vi "UI Initialize Device.vi"(8 "error in":errorcluster) -> (0 "error out":errorcluster)   [LabVIEW 2019, in "Initialize.lvlib"]
uses:
  Initialize.lvlib
  Queues/Message Cluster.ctl
  <vilib>/Utility/miscctls.llb/LVPointTypeDef.ctl
  Fluidic Process/SubVI/Fluidic Para.ctl
  LED/SubVI/Image Para.ctl
  Camera/Andor/SubVI/seletion.ctl
  <vilib>/Utility/file.llb/Read Delimited Spreadsheet (string).vi
  <vilib>/Utility/error.llb/Error Cluster From Error Code.vi
  <vilib>/ErrorRing/Error Ring.xnode
  Camera/Andor/Andor.lvlib
  IO/sbRIO9623/sbRIO9623.lvlib
  Laser/Coherent/Coherent.lvlib
  LED/LED.lvlib
  Motion/Allmotion/Allmotion.lvlib
  Selection Valve/IDEX/IDEX.lvlib
  Syringe Pump/NE-500/NE-500.lvlib
  Queues/Queues.lvlib
  Fluidic Process/Fluidic Process.lvlib
  Image/Image.lvlib
panel:
  in  "Start":bool
  in  "Operator":string
  in  "Experiment":string
  out "Homing":bool
  in  "Done":bool
  out "Syringe Pump":bool
  out "Selection Valve":bool
  out "Motion":bool
  out "LED":bool
  out "Laser":bool
  out "I/O":bool
  out "Camera":bool
  in  "Abort":bool
  in  "Next":bool
  # "Step 1. Experiment Info"
  # "Step 2. Device"
  # "Step 3. Chip"
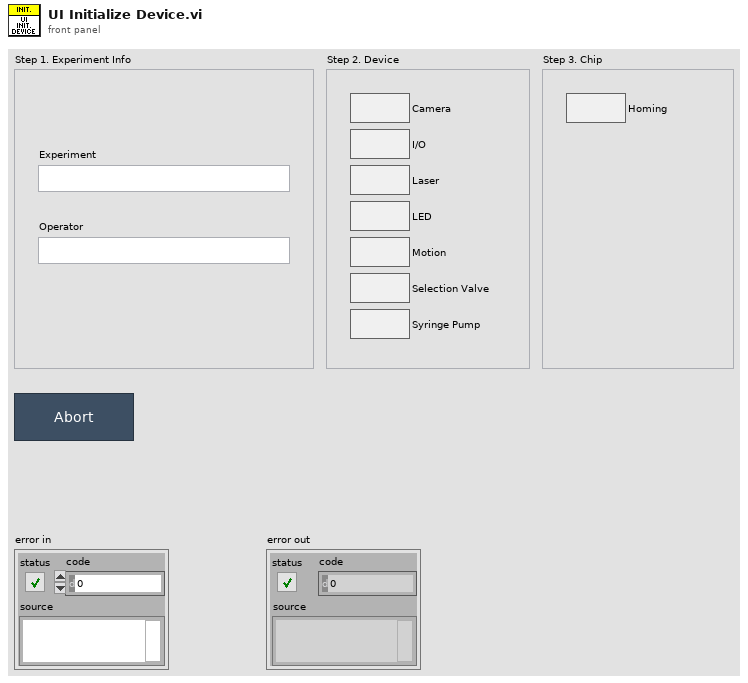
[diagram p1: front panel]
types:
  T1 = cluster{"VISA laser":refnum<visa-resource-name>, "VISA motion":refnum<visa-resource-name>, "Device Status":cluster{"Syringe Pump":bool, "Selection Valve":bool, "Motion":bool, "Camera":bool, "LED":bool, "Laser":bool, "I/O":bool}, "Tick Count":u32, "Chip Status":cluster{"Air Sealing":bool, "Homing":bool, "Locating":bool}, "Experiment":string, "Operator":string, "Folder Path":path}
  T2 = typedef "LVPointTypeDef.ctl" = cluster{"Horizontal":i16, "Vertical":i16}
  T3 = typedef "Queues.lvlib/Message Cluster.ctl" = cluster{"State":string, "Data":variant}
  T4 = typedef "Fluidic Process.lvlib/Fluidic Para.ctl" = cluster{"Read Force Sensor":i32, "Read Regulator":i32, "Read Force Sensor?":bool, "Read Regulator?":bool, "Read Syringe Pump":i32, "Read Syringe Pump?":bool}
  T5 = typedef "LED.lvlib/Image Para.ctl" = cluster{"Marker":T6, "Power(Amp)":u8, "set shutter(s)":dbl, "Cube":enum16{"1", "2", "3", "4", "5", "6", "7", "8"}}
  T6 = typedef "Andor.lvlib/seletion.ctl" = enum16{"None", "Red", "Green", "Blue", "UV", "Green Laser", "Blue-Red", "UV-Red", "BF", "UV-IR"}
  T7 = typedef "ROI Descriptor" = cluster{"Global Rectangle":i32[], "Contours":cluster{"ID":enum32{"External", "Internal"}, "Type":u32, "Coordinates":i32[]}[]}
  T8 = cluster{"Image Path":path, "Start Offset":i32, "Template Path":path, "Disable Fine Search":bool, "ROI":T7}
  T9 = typedef "Initialize.lvlib/SEQ Data.ctl" = cluster{"Folder Path":path}
  T10 = typedef "Andor.lvlib/SEQ Data.ctl" = cluster{"Initialize Sucess?":bool, "Image Ref":T11, "VI Refnum":refnum<vi>}
  T11 = typedef "IMAQ Image.ctl" = refnum<image>
  T12 = typedef "sbRIO9623.lvlib/SEQ Data.ctl" = cluster{"Lid Sensor 1":bool, "Lid Sensor 2":bool, "Laser Interlock":bool, "Buffer Tank":bool, "Wash Tank":bool, "Waste Tank":bool, "SiPM 1":fxp<+,20,5>, "SiPM 2":fxp<+,20,5>, "Initialize Success?":bool, "VI Refnum":refnum<vi>}
  T13 = typedef "Coherent.lvlib/SEQ Data.ctl" = cluster{"Initialize Success?":bool, "VI Refnum":refnum<vi>}
  T14 = typedef "LED.lvlib/SEQ Data.ctl" = cluster{"Initialize Sucess?":bool, "BL2 Regulator":dbl, "BL1 Regulator":dbl, "Blood Sensor 1":dbl, "Blood Sensor 2":dbl, "Air Pressure Sensor":dbl, "Force Snesor 1":u32, "Force Snesor 2":u32, "VI Refnum":refnum<vi>}
  T15 = typedef "Allmotion.lvlib/SEQ Data.ctl" = cluster{"Position":i32[], "Arrived?":bool, "VISA name":refnum<visa-resource-name>, "Initialize Done?":bool, "State":string, "VI Refnum":refnum<vi>, "Dichroic Position":string[]}
  T16 = typedef "IDEX.lvlib/SEQ Data.ctl" = cluster{"Position":string, "Initialize Done?":bool, "VI Refnum":refnum<vi>}
  T17 = typedef "NE-500.lvlib/SEQ Data.ctl" = cluster{"Status":string, "Initialize Done?":bool, "VI Refnum":refnum<vi>}
  T18 = typedef "Fluidic Process.lvlib/SEQ Data.ctl" = cluster{"Fluidic Process Done?":bool, "Current Process":i32, "Remaining Time":dbl, "Total Process":i32, "Air Sealing":bool, "Force Condition":bool}
  T19 = typedef "Rendezvous RefNum" = refnum<k1>
  T20 = typedef "Image.lvlib/SEQ Data.ctl" = cluster{"Acquire Done?":bool, "Focus Done?":bool, "Align Done?":bool, "No Position Match?":bool, "Best Wheel Position":string, "Match Done?":bool, "Match Score":dbl, "Focus Score":dbl, "Match Position":cluster{"x":sgl, "y":sgl}, "Flower Position":i32[]}
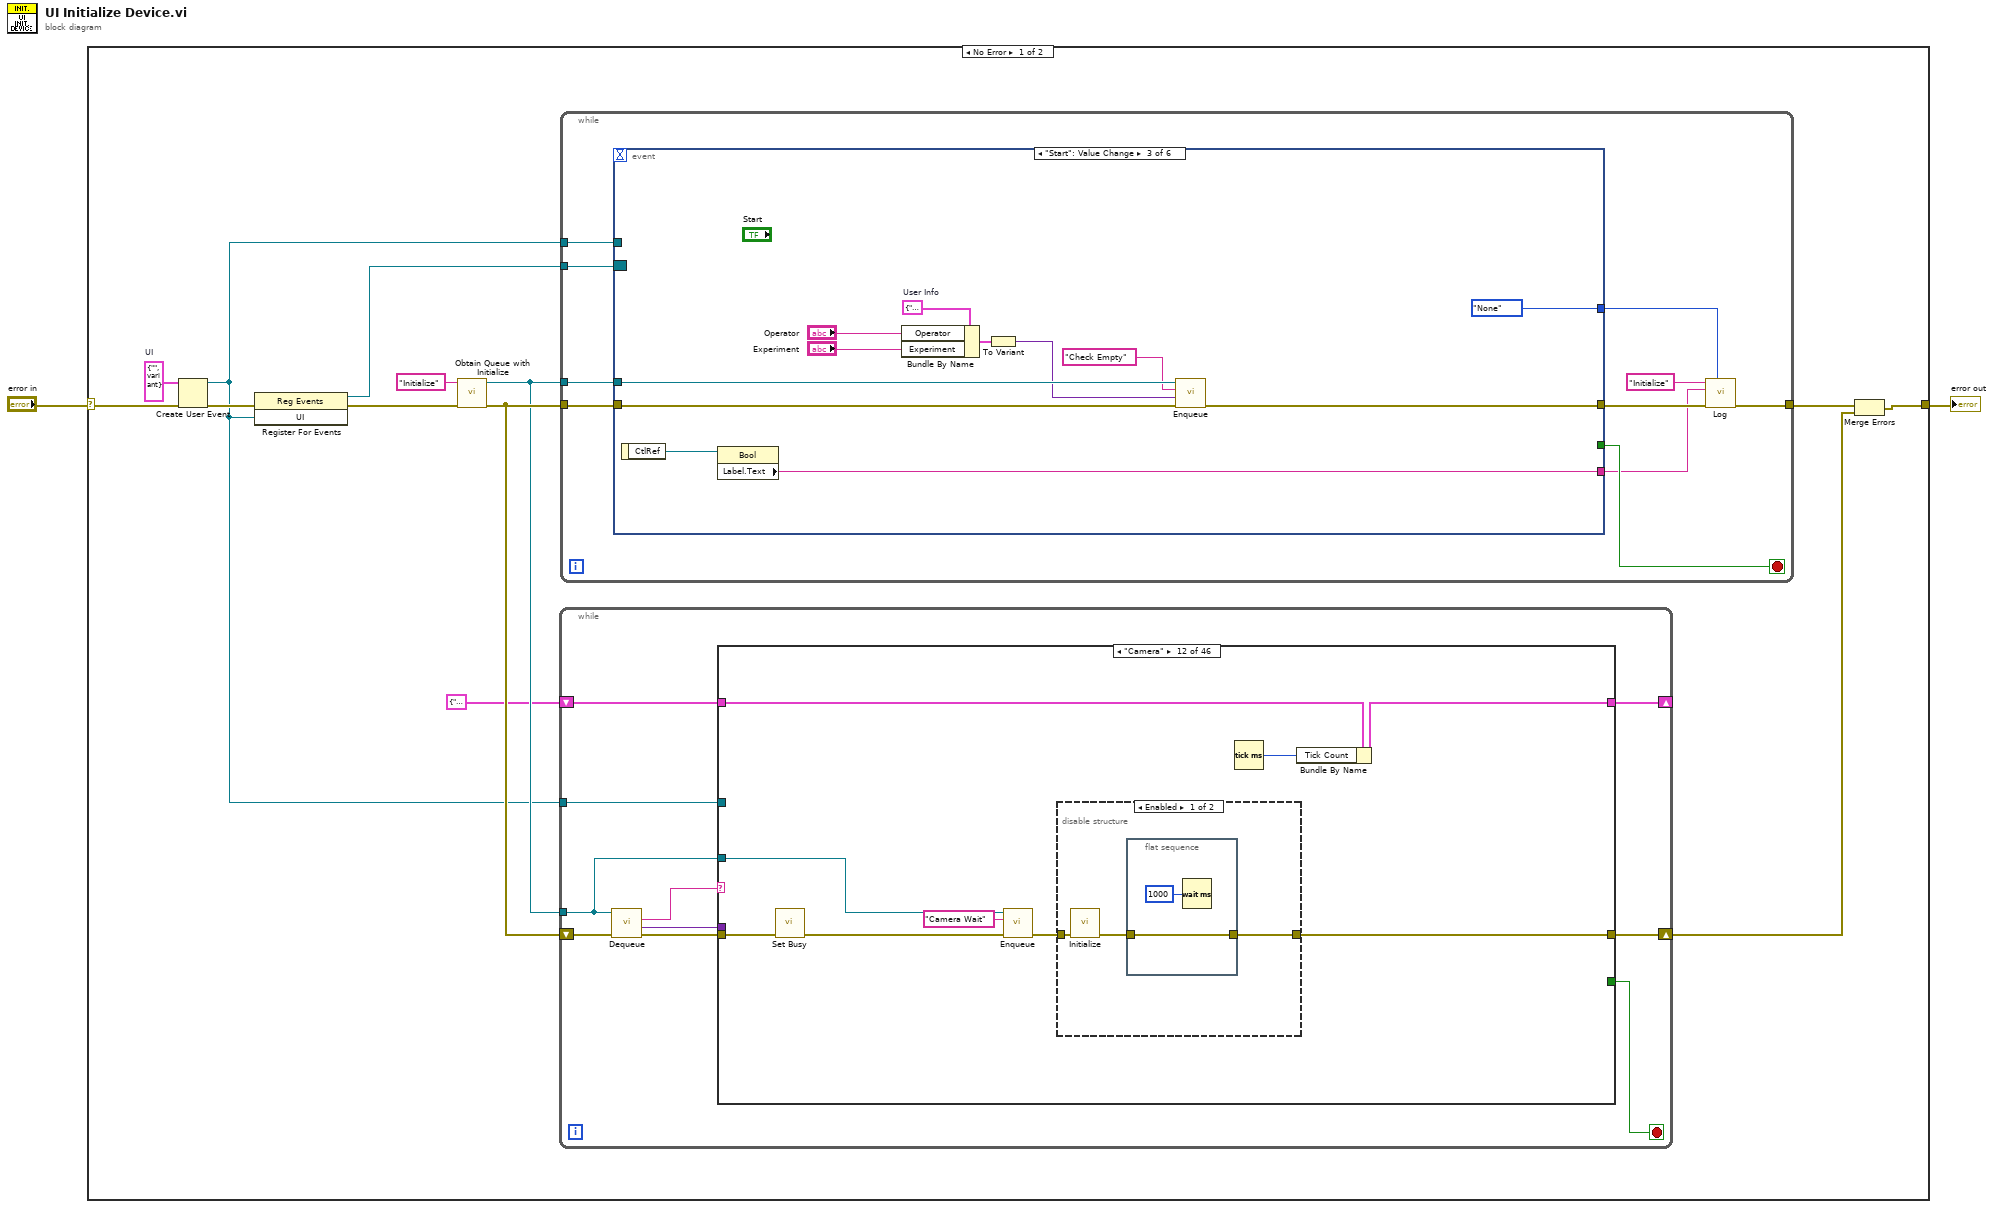
[diagram p0: block diagram]
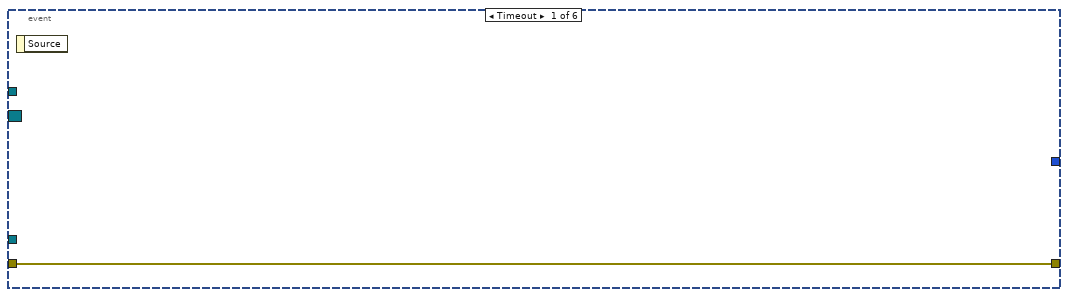
[diagram p2: hidden frame]
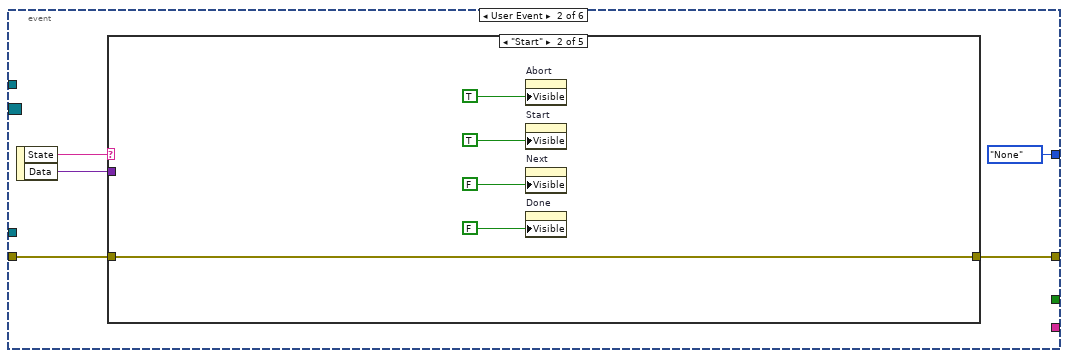
[diagram p3: hidden frame]
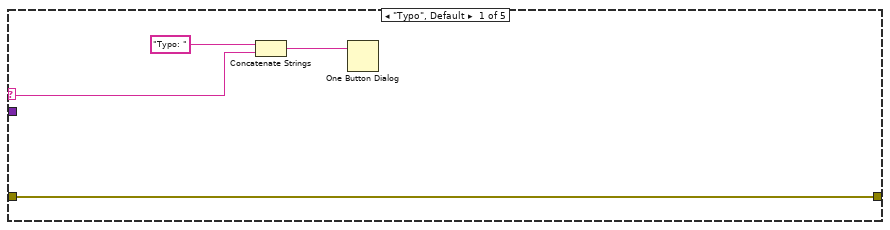
[diagram p4: hidden frame]
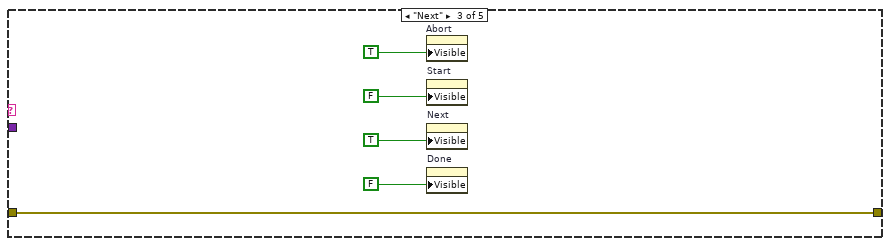
[diagram p5: hidden frame]
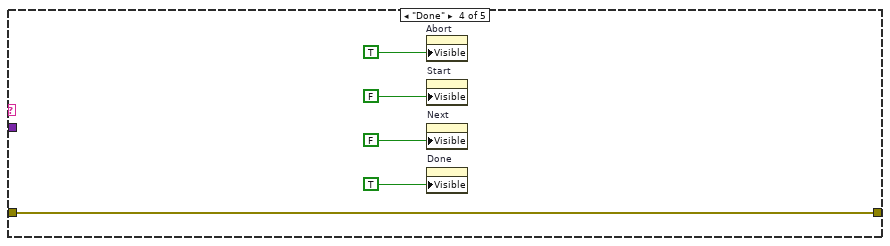
[diagram p6: hidden frame]
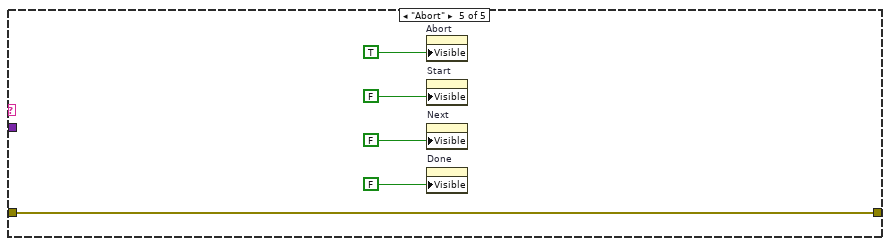
[diagram p7: hidden frame]
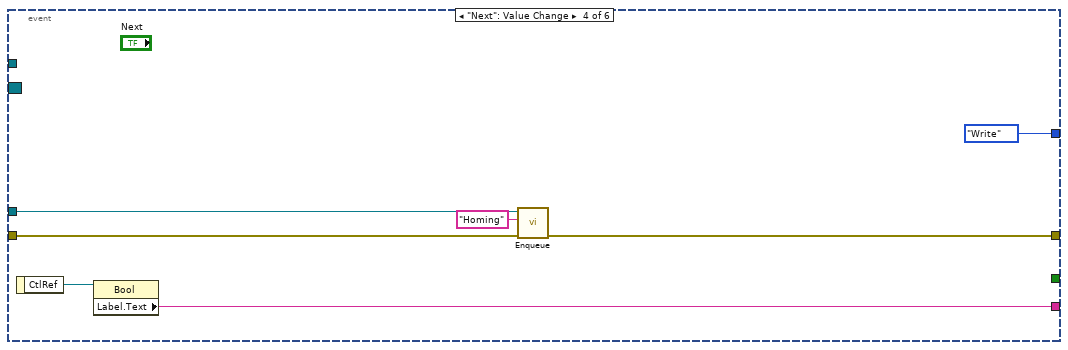
[diagram p8: hidden frame]
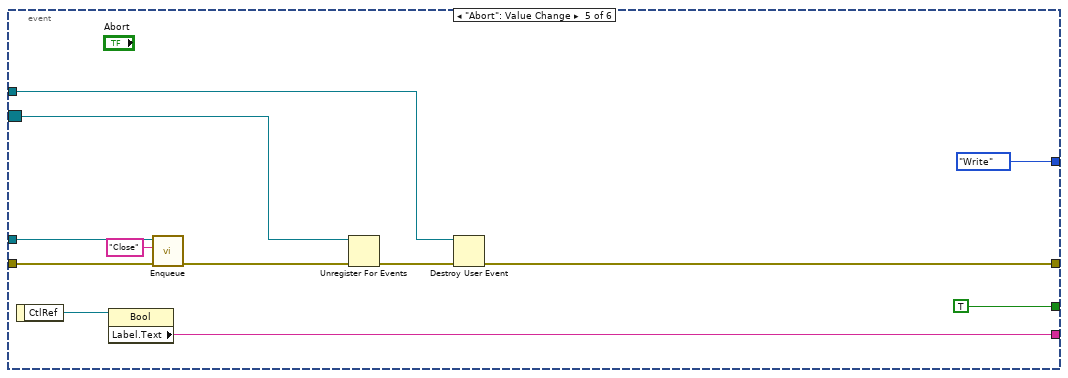
[diagram p9: hidden frame]
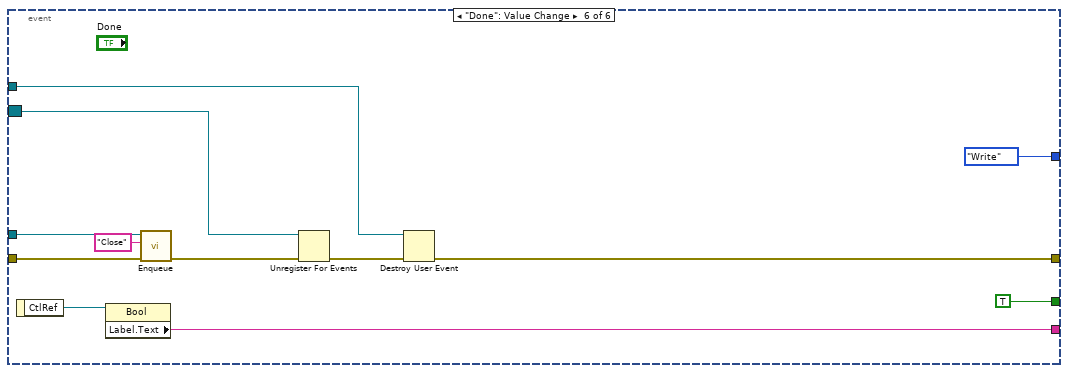
[diagram p10: hidden frame]
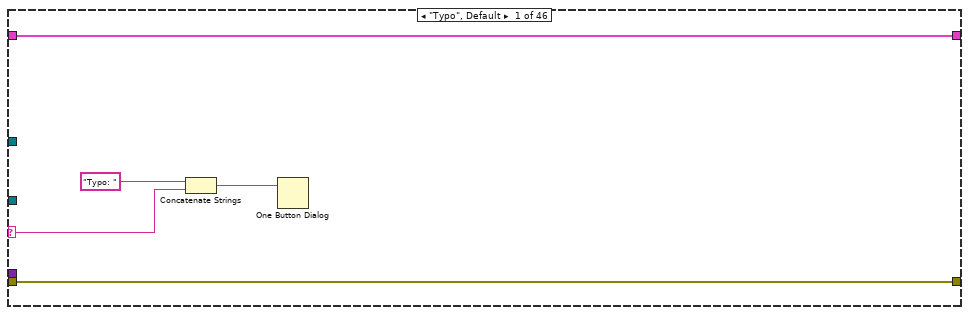
[diagram p11: hidden frame]
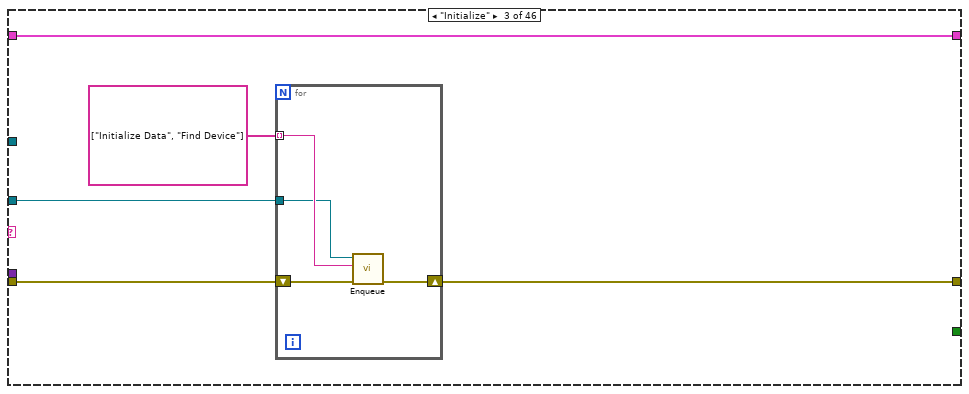
[diagram p13: hidden frame]
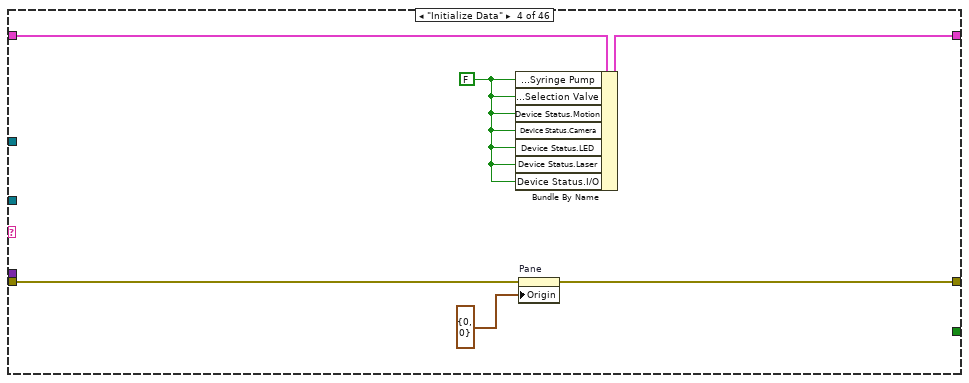
[diagram p14: hidden frame]
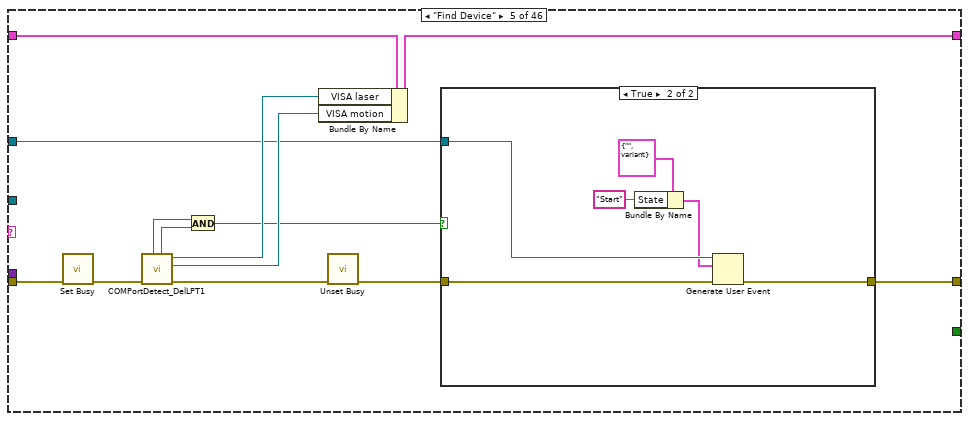
[diagram p15: hidden frame]
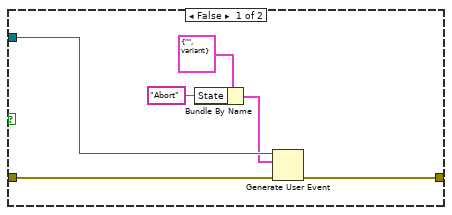
[diagram p16: hidden frame]
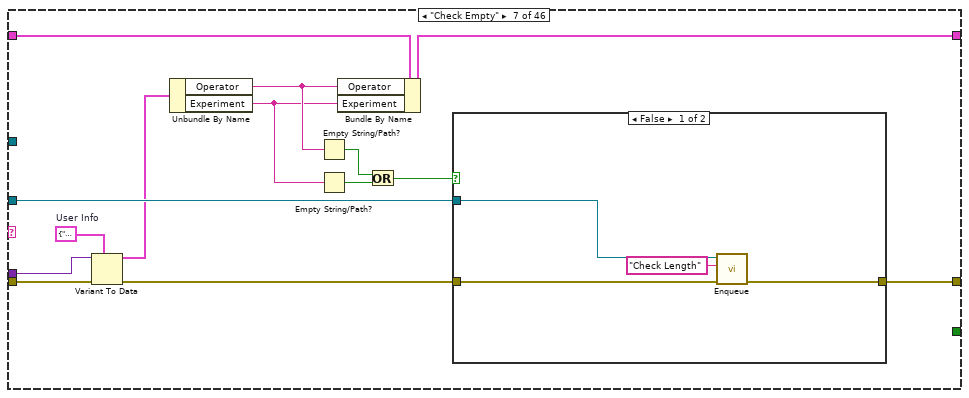
[diagram p18: hidden frame]
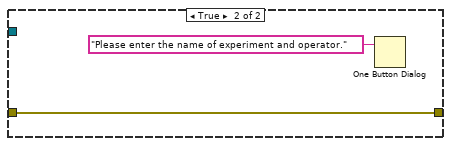
[diagram p19: hidden frame]
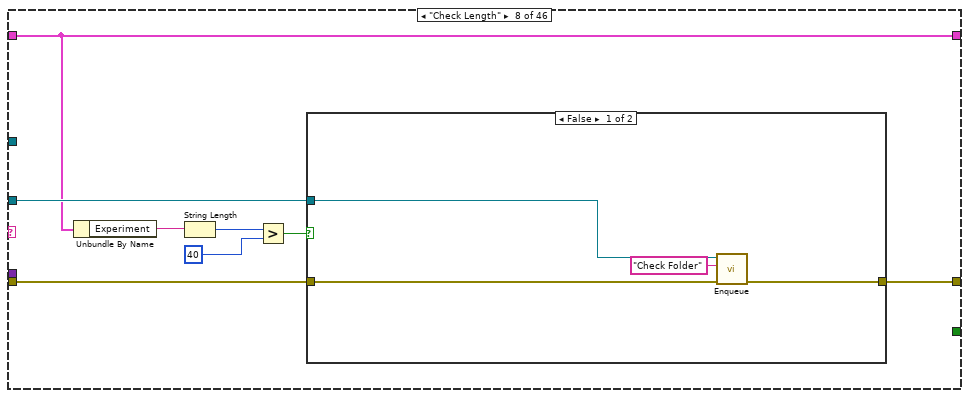
[diagram p20: hidden frame]
diagram:
  n1 = case shown="No Error" "error in" {
    selector: "error in" -> [w15 w771]
    tunnel: [w6 w771] -> w1
    frame No Error {
      w13 = T3 {"State"="", "Data"=variant}  # UI
      n2 = Create User Event(user event datatype=w13, error in=w15) -> (user event=w3:refnum<user-event>, error out=w14:errorcluster)
      n3 = register-events(error in=w14, w3) -> (reference out=w4:refnum<event-registration>, error out=w10:errorcluster)  [unwired: 1 in]
      n4 = call "Obtain Queue with Initialize.vi"("Error In"=w10, "Queue Name"="Initialize") -> ("Error Out"=w9:errorcluster, "Queue out"=w7:refnum<queue>)  [unwired: 8 in]
      n5 = while {
        tunnel: w7 -> [w104]
        shift-right: [w103] -> w11
        shift-left: w9 -> [w108]
        shift-right: [w100] -> _
        shift-left: T1 {"VISA laser"="", "VISA motion"="", "Device Status"={"Syringe Pump"=FALSE, "Selection Valve"=FALSE, "Motion"=FALSE, "Camera"=FALSE, "LED"=FALSE, "Laser"=FALSE, "I/O"=FALSE}, "Tick Count"=0, "Chip Status"={"Air Sealing"=FALSE, "Homing"=FALSE, "Locating"=FALSE}, "Experiment"="", "Operator"="", "Folder Path"=path ""} -> [w101]
        tunnel: w3 -> [w99]
        stop <- w102 stop-if-true
        n6 = call "Dequeue.vi"("Error In"=w108, "Queue in"=w104) -> ("Error Out"=w105:errorcluster, "Data"=w106:variant, "State"=w107:string)  [unwired: 6 in, 1 out]
        n7 = case shown="\"Camera\"" w107 {
          selector: w107 -> [w110 _ _ _ _ _ _ _ _ _ _ _ _ _ _ _ _ _ _ _ _ _ _ _ _ _ _ _ _ _ _ _ _ _ _ _ _ _ _ _ _ _ _ _ _ _]
          tunnel: w106 -> [_ _ _ _ _ _ w162 _ _ _ _ _ _ _ _ _ _ _ _ _ _ _ _ _ _ _ _ _ _ _ _ _ _ _ _ _ _ _ _ _ _ _ _ _ _ _]
          tunnel: w105 -> [w113 w114 w120 w127 w140 w156 w164 w183 w201 w232 w233 w236 w263 w283 w290 w317 w323 w349 w355 w382 w388 w415 w421 w448 w453 w470 w494 w503 w538 w543 w556 w578 w586 w594 w598 w629 w636 w664 w675 w704 w715 w737 w743 w747 w764 w770]
          tunnel: w104 -> [_ _ w117 _ _ _ w170 w181 w198 w231 _ w240 w254 w282 w294 w313 w327 w348 w359 w381 w392 w414 w425 w447 w457 w471 _ w501 w536 w551 w567 w577 w585 w593 w596 w628 w645 w663 w684 w703 w724 w736 w742 _ _ w769]
          tunnel: [w113 w114 w119 w126 w132 w156 w171 w182 w194 w228 w233 w242 w255 w278 w295 w314 w328 w344 w360 w375 w393 w406 w426 w439 w458 w473 w494 w498 w537 w546 w568 w572 w580 w588 w597 w624 w646 w665 w685 w705 w711 w730 w739 w750 w764 w768] -> w103
          tunnel: [_ _ _ _ _ _ _ _ _ _ _ _ _ _ _ _ _ _ _ _ _ _ _ _ _ _ _ _ _ _ _ _ _ _ _ _ _ _ _ _ _ _ _ _ _ TRUE] -> w102
          tunnel: w101 -> [w109 w115 w116 w130 w143 w157 w169 w179 w200 w224 w234 w243 w262 w280 w301 w309 w334 w341 w366 w374 w399 w410 w432 w443 w465 w481 w495 w506 w535 w549 w566 w579 w587 w595 w608 w630 w633 w659 w672 w698 w712 w738 w744 w748 w765 w766]
          tunnel: [w109 w115 w116 w129 w137 w157 w168 w179 w193 w224 w234 w238 w253 w277 w293 w311 w326 w343 w358 w379 w391 w412 w424 w445 w456 w481 w495 w497 w528 w545 w560 w579 w587 w595 w608 w623 w633 w661 w672 w701 w712 w729 w744 w748 w765 w766] -> w100
          tunnel: w99 -> [_ _ _ _ w131 _ _ _ _ _ _ _ _ _ _ _ _ _ _ _ _ _ _ _ _ w469 _ _ _ _ _ _ _ _ _ _ _ _ _ _ _ _ _ w749 _ _]
          frame "Typo", Default {
            n8 = Concatenate Strings("Typo: " ("string"), w110) -> (w112:string)
            n9 = One Button Dialog(message=w112) -> ()  [unwired: 1 in, 1 out]
          }
          frame "------Initialize------" {
          }
          frame "Initialize" {
            n10 = for {
              shift-right: [w123] -> w119
              shift-left: w120 -> [w124]
              tunnel: string[] ["Initialize Data", "Find Device"] -> [w122] mode=indexing
              tunnel: w117 -> [w121]
              n11 = call "Enqueue.vi"("Error In"=w124, "State"=w122, "Queue in"=w121) -> ("Error Out"=w123:errorcluster)  [unwired: 7 in, 1 out]
            }
          }
          frame "Initialize Data" {
            w128 = FALSE ("Initial Status.Syringe Pump")
            n12 = Bundle By Name(cluster=w130, "Device Status.Syringe Pump"=w128, "Device Status.Selection Valve"=w128, "Device Status.Motion"=w128, "Device Status.Camera"=w128, "Device Status.LED"=w128, "Device Status.Laser"=w128, "Device Status.I/O"=w128) -> (w129:T1)
            n13 = property on="Pane" class="Pane"(error in=w127, "Origin"=T2 {"Horizontal"=0, "Vertical"=0}) -> (error out=w126:errorcluster)  [unwired: 1 in, 1 out]
          }
          frame "Find Device" {
            n14 = call <vilib>:"Set Busy.vi"("error in (no error)"=w140) -> ("error out"=w139:errorcluster)  [unwired: 9 in, 1 out]
            n15 = call "COMPortDetect_DelLPT1.vi"("error in"=w139) -> ("error out"=w138:errorcluster, "VISA motion"=w135:refnum<visa-resource-name>, "VISA laser"=w136:refnum<visa-resource-name>, "Motion Find?"=w142:bool, "Laser Find?"=w141:bool)  [unwired: 6 in]
            n16 = And(x=w141, y=w142) -> (x .and. y?=w134:bool)
            n17 = Bundle By Name(cluster=w143, "VISA laser"=w136, "VISA motion"=w135) -> (w137:T1)
            n18 = call <vilib>:"Unset Busy.vi"("error in (no error)"=w138) -> ("error out"=w133:errorcluster)  [unwired: 10 in]
            n19 = case shown="True" w134 {
              tunnel: w133 -> [w149 w155]
              tunnel: [w148 w151] -> w132
              tunnel: w131 -> [w147 w154]
              frame False {
                n20 = Bundle By Name(cluster=T3 {"State"="", "Data"=variant} ("event data"), "State"="Abort") -> (w145:T3)
                n21 = Generate User Event(user event=w147, event data cluster=w145, error in=w149) -> (error out=w148:errorcluster)  [unwired: 1 in, 1 out]
              }
              frame True {
                n22 = Bundle By Name(cluster=T3 {"State"="", "Data"=variant} ("event data"), "State"="Start") -> (w152:T3)
                n23 = Generate User Event(user event=w154, event data cluster=w152, error in=w155) -> (error out=w151:errorcluster)  [unwired: 1 in, 1 out]
              }
            }
          }
          frame "------Create Folder------" {
          }
          frame "Check Empty" {
            w161 = cluster{"Operator":string, "Experiment":string} {"Operator"="", "Experiment"=""}  # User Info
            n24 = Variant To Data(error in=w164, type=w161, Variant=w162) -> (data=w160:cluster{"Operator":string, "Experiment":string}, error out=w163:errorcluster)
            n25 = Unbundle By Name(w160) -> ("Operator"=w159:string, "Experiment"=w158:string)
            n26 = Empty String/Path?(string/path=w159) -> (empty?=w167:bool)
            n27 = Empty String/Path?(string/path=w158) -> (empty?=w166:bool)
            n28 = Bundle By Name(cluster=w169, "Operator"=w159, "Experiment"=w158) -> (w168:T1)
            n29 = Or(x=w167, y=w166) -> (x .or. y?=w165:bool)
            n30 = case shown="False" w165 {
              tunnel: w163 -> [w175 w177]
              tunnel: [w174 w177] -> w171
              tunnel: w170 -> [w173 _]
              frame False {
                n31 = call "Enqueue.vi"("Error In"=w175, "State"="Check Length", "Queue in"=w173) -> ("Error Out"=w174:errorcluster)  [unwired: 7 in, 1 out]
              }
              frame True {
                n32 = One Button Dialog(message="Please enter the name of experiment and operator.") -> ()  [unwired: 1 in, 1 out]
              }
            }
          }
          frame "Check Length" {
            n33 = Unbundle By Name(w179) -> ("Experiment"=w178:string)
            n34 = String Length(string=w178) -> (length=w185:i32)
            n35 = Greater?(x=w185, y=40) -> (0:w180:bool)
            n36 = case shown="False" w180 {
              tunnel: w183 -> [w189 w191]
              tunnel: [w188 w191] -> w182
              tunnel: w181 -> [w187 _]
              frame False {
                n37 = call "Enqueue.vi"("Error In"=w189, "State"="Check Folder", "Queue in"=w187) -> ("Error Out"=w188:errorcluster)  [unwired: 7 in, 1 out]
              }
              frame True {
                n38 = One Button Dialog(message="Please limit the Sample ID to less than 40 characters and do not use spaces and symbols.") -> ()  [unwired: 1 in, 1 out]
              }
            }
          }
          frame "Check Folder" {
            n39 = Unbundle By Name(w200) -> ("Experiment"=w199:string)
            n40 = Format Date/Time String(time format string (%c)="%Y%m%d") -> (date/time string=w205:string)  [unwired: 2 in]
            n41 = Concatenate Strings(w205, "\\", w199) -> (w206:string)
            n42 = Build Path(base path=path "C:/MiCareo/MiSelect2015QQ01/DATA", name or relative path=w206) -> (appended path=w207:path)
            n43 = call <vilib>:"Check if File or Folder Exists.vi"("error in (no error)"=w201, "path"=w207) -> ("error out"=w195:errorcluster, "file or folder exists?"=w197:bool, "dup path"=w196:path)  [unwired: 7 in]
            n44 = case shown="False" w197 {
              tunnel: w198 -> [w215 _]
              tunnel: w196 -> [w208 _]
              tunnel: w195 -> [w217 w219]
              tunnel: [w216 w219] -> w194
              tunnel: [w208 _] -> w192
              frame False {
                n45 = Create Folder(path (use dialog)=w208, error in=w217) -> (error out=w213:errorcluster)  [unwired: 1 in, 2 out]
                n46 = call "SEQ Preview Queue.vi"("error in"=w213) -> ("error out"=w212:errorcluster, "SEQ Data"=w210:T9)  [unwired: 9 in]
                n47 = Bundle By Name(cluster=w210, "Folder Path"=w208) -> (w209:T9)
                n48 = call "SEQ Lossy Queue.vi"("error in"=w212, "SEQ Data"=w209) -> ("error out"=w211:errorcluster)  [unwired: 9 in]
                n49 = call "Enqueue.vi"("Error In"=w211, "State"="Write User Info", "Queue in"=w215) -> ("Error Out"=w216:errorcluster)  [unwired: 7 in, 1 out]
              }
              frame True {
                n50 = One Button Dialog(message="This name of the experiment has already been used") -> ()  [unwired: 1 in, 1 out]
              }
            }
            n51 = Bundle By Name(cluster=w200, "Folder Path"=w192) -> (w193:T1)
          }
          frame "Write User Info" {
            n52 = Unbundle By Name(w224) -> ("Operator"=w222:string, "Experiment"=w221:string)
            n53 = call "Enqueue.vi"("Error In"=w232, "State"="Camera", "Queue in"=w231) -> ("Error Out"=w229:errorcluster)  [unwired: 7 in, 1 out]
            n54 = Format Into String(format string="Operator: %s, Experiment: %s", w222, w221) -> (resulting string=w220:string)  [unwired: 2 in, 1 out]
            n55 = call "Log.vi"("Action"=enum16{"None", "Write"}."Write", "error in"=w229, "Description"=w220, "State"="User Info", "Page Name"="Initialize") -> ("error out"=w228:errorcluster)  [unwired: 6 in]
          }
          frame "------Device------" {
          }
          frame "Camera" {
            n56 = call <vilib>:"Set Busy.vi"("error in (no error)"=w236) -> ("error out"=w235:errorcluster)  [unwired: 9 in, 1 out]
            n57 = call "Enqueue.vi"("Error In"=w235, "State"="Camera Wait", "Queue in"=w240) -> ("Error Out"=w241:errorcluster)  [unwired: 7 in, 1 out]
            n58 = disable-structure shown="Enabled" {
              disable-tunnel: [w245 w249] -> w242
              disable-tunnel: w241 -> [w244 w249]
              frame Enabled {
                n59 = call "Initialize.vi"("Error In"=w244) -> ("Error Out"=w246:errorcluster)  [unwired: 10 in]
                n60 = flat-sequence {
                  tunnel: w246 -> [w247]
                  tunnel: [w247] -> w245
                  frame #0 {
                    n61 = Wait (ms)(milliseconds to wait=u32 1000) -> ()  [unwired: 1 out]
                  }
                }
              }
              frame Disabled {
              }
            }
            n62 = Tick Count (ms)() -> (millisecond timer value=w237:u32)
            n63 = Bundle By Name(cluster=w243, "Tick Count"=w237) -> (w238:T1)
          }
          frame "Camera Wait" {
            n64 = disable-structure shown="Enabled" {
              disable-tunnel: w263 -> [w267 w270]
              disable-tunnel: [w266 w270] -> w256
              disable-tunnel: [w265 TRUE ("Camera")] -> w252
              frame Enabled {
                n65 = call "SEQ Preview Queue.vi"("error in"=w267) -> ("error out"=w266:errorcluster, "SEQ Data"=w268:T10)  [unwired: 9 in]
                n66 = Unbundle By Name(w268) -> ("Initialize Sucess?"=w265:bool)
              }
              frame Disabled {
              }
            }
            "Camera" <- w252
            n67 = Unbundle By Name(w262) -> ("Tick Count"=w260:u32)
            n68 = Tick Count (ms)() -> (millisecond timer value=w261:u32)
            n69 = Subtract(x=w261, y=w260) -> (x-y=w259:u32)
            n70 = Greater Or Equal?(x=w259, y=u32 15000) -> (x >= y?=w250:bool)
            n71 = Or(x=w250, y=w252) -> (x .or. y?=w257:bool)
            n72 = Wait (ms)(milliseconds to wait=u32 100) -> ()  [unwired: 1 out]
            n73 = Bundle By Name(cluster=w262, "Device Status.Camera"=w252) -> (w253:T1)
            n74 = case shown="True" w257 {
              tunnel: ["Camera Wait" w273] -> w251
              tunnel: w250 -> [_ w272]
              frame False {
              }
              frame True {
                n75 = case shown="True" w272 {
                  tunnel: ["I/O" "Device End"] -> w273
                  frame False {
                  }
                  frame True {
                  }
                }
              }
            }
            n76 = call "Enqueue.vi"("Error In"=w256, "State"=w251, "Queue in"=w254) -> ("Error Out"=w255:errorcluster)  [unwired: 7 in, 1 out]
          }
          frame "I/O" {
            n77 = call "Enqueue.vi"("Error In"=w283, "State"="I/O Wait", "Queue in"=w282) -> ("Error Out"=w279:errorcluster)  [unwired: 7 in, 1 out]
            n78 = call "Initialize.vi"("Error In"=w279) -> ("Error Out"=w284:errorcluster)  [unwired: 10 in]
            n79 = flat-sequence {
              tunnel: w284 -> [w285]
              tunnel: [w285] -> w278
              frame #0 {
                n80 = Wait (ms)(milliseconds to wait=u32 1000) -> ()  [unwired: 1 out]
              }
            }
            n81 = Tick Count (ms)() -> (millisecond timer value=w276:u32)
            n82 = Bundle By Name(cluster=w280, "Tick Count"=w276) -> (w277:T1)
          }
          frame "I/O Wait" {
            n83 = call "SEQ Preview Queue.vi"("error in"=w290) -> ("error out"=w289:errorcluster, "SEQ Data"=w291:T12)  [unwired: 9 in]
            n84 = Unbundle By Name(w301) -> ("Tick Count"=w299:u32)
            n85 = Unbundle By Name(w291) -> ("Initialize Success?"=w288:bool)
            "I/O" <- w288
            n86 = Tick Count (ms)() -> (millisecond timer value=w300:u32)
            n87 = Subtract(x=w300, y=w299) -> (x-y=w298:u32)
            n88 = Greater Or Equal?(x=w298, y=u32 15000) -> (x >= y?=w287:bool)
            n89 = Or(x=w287, y=w288) -> (x .or. y?=w296:bool)
            n90 = Wait (ms)(milliseconds to wait=u32 100) -> ()  [unwired: 1 out]
            n91 = Bundle By Name(cluster=w301, "Device Status.I/O"=w288) -> (w293:T1)
            n92 = case shown="True" w296 {
              tunnel: ["I/O Wait" w305] -> w292
              tunnel: w287 -> [_ w304]
              frame False {
              }
              frame True {
                n93 = case shown="True" w304 {
                  tunnel: ["Laser" "Device End"] -> w305
                  frame False {
                  }
                  frame True {
                  }
                }
              }
            }
            n94 = call "Enqueue.vi"("Error In"=w289, "State"=w292, "Queue in"=w294) -> ("Error Out"=w295:errorcluster)  [unwired: 7 in, 1 out]
          }
          frame "Laser" {
            n95 = Unbundle By Name(w309) -> ("VISA laser"=w308:refnum<visa-resource-name>)
            n96 = call "Enqueue.vi"("Error In"=w317, "State"="Laser Wait", "Queue in"=w313) -> ("Error Out"=w315:errorcluster)  [unwired: 7 in, 1 out]
            n97 = call "Initialize.vi"("Error In"=w315, "VISA in"=w308) -> ("Error Out"=w316:errorcluster)  [unwired: 9 in]
            n98 = flat-sequence {
              tunnel: w316 -> [w318]
              tunnel: [w318] -> w314
              frame #0 {
                n99 = Wait (ms)(milliseconds to wait=u32 1000) -> ()  [unwired: 1 out]
              }
            }
            n100 = Tick Count (ms)() -> (millisecond timer value=w310:u32)
            n101 = Bundle By Name(cluster=w309, "Tick Count"=w310) -> (w311:T1)
          }
          frame "Laser Wait" {
            n102 = call "SEQ Preview Queue.vi"("error in"=w323) -> ("error out"=w322:errorcluster, "SEQ Data"=w324:T13)  [unwired: 9 in]
            n103 = Unbundle By Name(w334) -> ("Tick Count"=w332:u32)
            n104 = Unbundle By Name(w324) -> ("Initialize Success?"=w321:bool)
            "Laser" <- w321
            n105 = Tick Count (ms)() -> (millisecond timer value=w333:u32)
            n106 = Subtract(x=w333, y=w332) -> (x-y=w331:u32)
            n107 = Greater Or Equal?(x=w331, y=u32 15000) -> (x >= y?=w320:bool)
            n108 = Or(x=w320, y=w321) -> (x .or. y?=w329:bool)
            n109 = Wait (ms)(milliseconds to wait=u32 100) -> ()  [unwired: 1 out]
            n110 = Bundle By Name(cluster=w334, "Device Status.Laser"=w321) -> (w326:T1)
            n111 = case shown="True" w329 {
              tunnel: ["Laser Wait" w338] -> w325
              tunnel: w320 -> [_ w337]
              frame False {
              }
              frame True {
                n112 = case shown="True" w337 {
                  tunnel: ["LED" "Device End"] -> w338
                  frame False {
                  }
                  frame True {
                  }
                }
              }
            }
            n113 = call "Enqueue.vi"("Error In"=w322, "State"=w325, "Queue in"=w327) -> ("Error Out"=w328:errorcluster)  [unwired: 7 in, 1 out]
          }
          frame "LED" {
            n114 = call "Enqueue.vi"("Error In"=w349, "State"="LED Wait", "Queue in"=w348) -> ("Error Out"=w345:errorcluster)  [unwired: 7 in, 1 out]
            n115 = call "Initialize.vi"("Error In"=w345) -> ("Error Out"=w346:errorcluster)  [unwired: 10 in]
            n116 = flat-sequence {
              tunnel: w346 -> [w350]
              tunnel: [w350] -> w344
              frame #0 {
                n117 = Wait (ms)(milliseconds to wait=u32 1000) -> ()  [unwired: 1 out]
              }
            }
            n118 = Tick Count (ms)() -> (millisecond timer value=w342:u32)
            n119 = Bundle By Name(cluster=w341, "Tick Count"=w342) -> (w343:T1)
          }
          frame "LED Wait" {
            n120 = call "SEQ Preview Queue.vi"("error in"=w355) -> ("error out"=w354:errorcluster, "SEQ Data"=w356:T14)  [unwired: 9 in]
            n121 = Unbundle By Name(w366) -> ("Tick Count"=w364:u32)
            n122 = Unbundle By Name(w356) -> ("Initialize Sucess?"=w353:bool)
            "LED" <- w353
            n123 = Tick Count (ms)() -> (millisecond timer value=w365:u32)
            n124 = Subtract(x=w365, y=w364) -> (x-y=w363:u32)
            n125 = Greater Or Equal?(x=w363, y=u32 15000) -> (x >= y?=w352:bool)
            n126 = Or(x=w352, y=w353) -> (x .or. y?=w361:bool)
            n127 = Wait (ms)(milliseconds to wait=u32 100) -> ()  [unwired: 1 out]
            n128 = Bundle By Name(cluster=w366, "Device Status.LED"=w353) -> (w358:T1)
            n129 = case shown="True" w361 {
              tunnel: ["LED Wait" w370] -> w357
              tunnel: w352 -> [_ w369]
              frame False {
              }
              frame True {
                n130 = case shown="True" w369 {
                  tunnel: ["Motion" "Device End"] -> w370
                  frame False {
                  }
                  frame True {
                  }
                }
              }
            }
            n131 = call "Enqueue.vi"("Error In"=w354, "State"=w357, "Queue in"=w359) -> ("Error Out"=w360:errorcluster)  [unwired: 7 in, 1 out]
          }
          frame "Motion" {
            n132 = Unbundle By Name(w374) -> ("VISA motion"=w373:refnum<visa-resource-name>)
            n133 = call "Enqueue.vi"("Error In"=w382, "State"="Motion Wait", "Queue in"=w381) -> ("Error Out"=w376:errorcluster)  [unwired: 7 in, 1 out]
            n134 = call "Initialize.vi"("Error In"=w376, "VISA in"=w373) -> ("Error Out"=w377:errorcluster)  [unwired: 9 in]
            n135 = flat-sequence {
              tunnel: w377 -> [w383]
              tunnel: [w383] -> w375
              frame #0 {
                n136 = Wait (ms)(milliseconds to wait=u32 1000) -> ()  [unwired: 1 out]
              }
            }
            n137 = Tick Count (ms)() -> (millisecond timer value=w378:u32)
            n138 = Bundle By Name(cluster=w374, "Tick Count"=w378) -> (w379:T1)
          }
          frame "Motion Wait" {
            n139 = call "SEQ Preview Queue.vi"("error in"=w388) -> ("error out"=w387:errorcluster, "SEQ Data"=w389:T15)  [unwired: 9 in]
            n140 = Unbundle By Name(w399) -> ("Tick Count"=w397:u32)
            n141 = Unbundle By Name(w389) -> ("Initialize Done?"=w386:bool)
            "Motion" <- w386
            n142 = Tick Count (ms)() -> (millisecond timer value=w398:u32)
            n143 = Subtract(x=w398, y=w397) -> (x-y=w396:u32)
            n144 = Greater Or Equal?(x=w396, y=u32 15000) -> (x >= y?=w385:bool)
            n145 = Or(x=w385, y=w386) -> (x .or. y?=w394:bool)
            n146 = Wait (ms)(milliseconds to wait=u32 100) -> ()  [unwired: 1 out]
            n147 = Bundle By Name(cluster=w399, "Device Status.Motion"=w386) -> (w391:T1)
            n148 = case shown="True" w394 {
              tunnel: ["Motion Wait" w403] -> w390
              tunnel: w385 -> [_ w402]
              frame False {
              }
              frame True {
                n149 = case shown="True" w402 {
                  tunnel: ["Selection Valve" "Device End"] -> w403
                  frame False {
                  }
                  frame True {
                  }
                }
              }
            }
            n150 = call "Enqueue.vi"("Error In"=w387, "State"=w390, "Queue in"=w392) -> ("Error Out"=w393:errorcluster)  [unwired: 7 in, 1 out]
          }
          frame "Selection Valve" {
            n151 = call "Enqueue.vi"("Error In"=w415, "State"="Selection Valve Wait", "Queue in"=w414) -> ("Error Out"=w407:errorcluster)  [unwired: 7 in, 1 out]
            n152 = call "Initialize.vi"("Error In"=w407, "VISA name"=refnum<visa-resource-name> "visa://169.254.25.118/ASRL1::INSTR") -> ("Error Out"=w409:errorcluster)  [unwired: 9 in]
            n153 = Tick Count (ms)() -> (millisecond timer value=w411:u32)
            n154 = flat-sequence {
              tunnel: w409 -> [w416]
              tunnel: [w416] -> w406
              frame #0 {
                n155 = Wait (ms)(milliseconds to wait=u32 1000) -> ()  [unwired: 1 out]
              }
            }
            n156 = Bundle By Name(cluster=w410, "Tick Count"=w411) -> (w412:T1)
          }
          frame "Selection Valve Wait" {
            n157 = call "SEQ Preview Queue.vi"("error in"=w421) -> ("error out"=w420:errorcluster, "SEQ Data"=w422:T16)  [unwired: 9 in]
            n158 = Unbundle By Name(w432) -> ("Tick Count"=w430:u32)
            n159 = Unbundle By Name(w422) -> ("Initialize Done?"=w419:bool)
            "Selection Valve" <- w419
            n160 = Tick Count (ms)() -> (millisecond timer value=w431:u32)
            n161 = Subtract(x=w431, y=w430) -> (x-y=w429:u32)
            n162 = Greater Or Equal?(x=w429, y=u32 15000) -> (x >= y?=w418:bool)
            n163 = Or(x=w418, y=w419) -> (x .or. y?=w427:bool)
            n164 = Wait (ms)(milliseconds to wait=u32 100) -> ()  [unwired: 1 out]
            n165 = Bundle By Name(cluster=w432, "Device Status.Selection Valve"=w419) -> (w424:T1)
            n166 = case shown="True" w427 {
              tunnel: ["Selection Valve Wait" w436] -> w423
              tunnel: w418 -> [_ w435]
              frame False {
              }
              frame True {
                n167 = case shown="True" w435 {
                  tunnel: ["Syringe Pump" "Device End"] -> w436
                  frame False {
                  }
                  frame True {
                  }
                }
              }
            }
            n168 = call "Enqueue.vi"("Error In"=w420, "State"=w423, "Queue in"=w425) -> ("Error Out"=w426:errorcluster)  [unwired: 7 in, 1 out]
          }
          frame "Syringe Pump" {
            n169 = call "Enqueue.vi"("Error In"=w448, "State"="Syringe Pump Wait", "Queue in"=w447) -> ("Error Out"=w440:errorcluster)  [unwired: 7 in, 1 out]
            n170 = call "Initialize.vi"("Error In"=w440, "VISA name"=refnum<visa-resource-name> "visa://169.254.25.118/ASRL2::INSTR") -> ("Error Out"=w442:errorcluster)  [unwired: 9 in]
            n171 = Tick Count (ms)() -> (millisecond timer value=w444:u32)
            n172 = flat-sequence {
              tunnel: w442 -> [w450]
              tunnel: [w450] -> w439
              frame #0 {
                n173 = Wait (ms)(milliseconds to wait=u32 1000) -> ()  [unwired: 1 out]
              }
            }
            n174 = Bundle By Name(cluster=w443, "Tick Count"=w444) -> (w445:T1)
          }
          frame "Syringe Pump Wait" {
            n175 = call "SEQ Preview Queue.vi"("error in"=w453) -> ("error out"=w452:errorcluster, "SEQ Data"=w454:T17)  [unwired: 9 in]
            n176 = Unbundle By Name(w465) -> ("Tick Count"=w463:u32)
            n177 = Unbundle By Name(w454) -> ("Initialize Done?"=w451:bool)
            "Syringe Pump" <- w451
            n178 = Tick Count (ms)() -> (millisecond timer value=w464:u32)
            n179 = Subtract(x=w464, y=w463) -> (x-y=w462:u32)
            n180 = Greater Or Equal?(x=w462, y=u32 15000) -> (x >= y?=w460:bool)
            n181 = Or(x=w460, y=w451) -> (x .or. y?=w459:bool)
            n182 = Wait (ms)(milliseconds to wait=u32 100) -> ()  [unwired: 1 out]
            n183 = Bundle By Name(cluster=w465, "Device Status.Syringe Pump"=w451) -> (w456:T1)
            n184 = case shown="True" w459 {
              tunnel: ["Syringe Pump Wait" "Device End"] -> w455
              frame False {
              }
              frame True {
              }
            }
            n185 = call "Enqueue.vi"("Error In"=w452, "State"=w455, "Queue in"=w457) -> ("Error Out"=w458:errorcluster)  [unwired: 7 in, 1 out]
          }
          frame "Device End" {
            n186 = Unbundle By Name(w481) -> ("Device Status.Syringe Pump"=w480:bool, "Device Status.Selection Valve"=w479:bool, "Device Status.Motion"=w478:bool, "Device Status.Camera"=w477:bool, "Device Status.LED"=w476:bool, "Device Status.Laser"=w475:bool, "Device Status.I/O"=w474:bool)
            n187 = Compound Arithmetic op=AND(w480, w479, w478, w477, w476, w475, w474) -> (w472:bool)
            n188 = case shown="False" w472 {
              tunnel: w470 -> [w489 w493]
              tunnel: [w482 w492] -> w473
              tunnel: w471 -> [_ w491]
              tunnel: w469 -> [w484 _]
              frame False {
                n189 = Bundle By Name(cluster=T3 {"State"="", "Data"=variant} ("event data"), "State"="Abort") -> (w487:T3)
                n190 = Generate User Event(user event=w484, event data cluster=w487, error in=w489) -> (error out=w483:errorcluster)  [unwired: 1 in, 1 out]
                n191 = call <vilib>:"Unset Busy.vi"("error in (no error)"=w483) -> ("error out"=w482:errorcluster)  [unwired: 10 in]
                n192 = One Button Dialog(message="Device Initialization Fail. Please Click \"Abort\".") -> ()  [unwired: 1 in, 1 out]
              }
              frame True {
                n193 = call "Enqueue.vi"("Error In"=w493, "State"="Homing", "Queue in"=w491) -> ("Error Out"=w492:errorcluster)  [unwired: 7 in, 1 out]
              }
            }
          }
          frame "------Chip------" {
          }
          frame "Air Tight" {
            w508 = 0 ("Read Force Sensor")
            w507 = FALSE ("Read Force Sensor?")
            n194 = call "Enqueue.vi"("Error In"=w503, "State"="Air Tight Wait", "Queue in"=w501) -> ("Error Out"=w502:errorcluster)  [unwired: 7 in, 1 out]
            n195 = call <vilib>:"Set Busy.vi"("error in (no error)"=w502) -> ("error out"=w505:errorcluster)  [unwired: 9 in, 1 out]
            n196 = Bundle By Name(cluster=T4 {"Read Force Sensor"=0, "Read Regulator"=0, "Read Force Sensor?"=FALSE, "Read Regulator?"=FALSE, "Read Syringe Pump"=0, "Read Syringe Pump?"=FALSE} ("Fluidic Para"), "Read Regulator"=2, "Read Regulator?"=TRUE, "Read Force Sensor"=w508, "Read Syringe Pump"=w508, "Read Force Sensor?"=w507, "Read Syringe Pump?"=w507) -> (w512:T4)
            n197 = disable-structure shown="RUN_TIME_ENGINE==True" {
              disable-tunnel: [w518 w521] -> w513
              frame condition #0 (active) {
                n198 = call <vilib>:"Application Directory.vi"() -> ("Application Directory"=w517:path)
                n199 = Build Path(base path=w517, name or relative path="Fluidic Process\\File\\Air Tight.txt") -> (appended path=w518:path)
              }
              frame condition #1 {
                n200 = call <vilib>:"Application Directory.vi"() -> ("Application Directory"=w520:path)
                n201 = Build Path(base path=w520, name or relative path="data\\File\\Air Tight.txt") -> (appended path=w521:path)
              }
            }
            n202 = call "Update Fluidic Para.vi"("Error In"=w505, "Fluidic Para"=w512) -> ("Error Out"=w504:errorcluster)  [unwired: 9 in]
            n203 = Tick Count (ms)() -> (millisecond timer value=w496:u32)
            n204 = Bundle By Name(cluster=w506, "Tick Count"=w496) -> (w497:T1)
            n205 = call-poly <vilib>:"Read Delimited Spreadsheet.vi"("file path (dialog if empty)"=w513, "error in (no error)"=w504) -> ("all rows"=w515:string[][], "error out"=w514:errorcluster)  [unwired: 8 in, 4 out]
            n206 = call "Run Process.vi"("Error In"=w514, "Fluidic Process in"=w515) -> ("Error Out"=w499:errorcluster)  [unwired: 9 in]
            n207 = flat-sequence {
              tunnel: w499 -> [w523]
              tunnel: [w523] -> w498
              frame #0 {
                n208 = Wait (ms)(milliseconds to wait=u32 1000) -> ()  [unwired: 1 out]
              }
            }
          }
          frame "Air Tight Wait" {
            n209 = Tick Count (ms)() -> (millisecond timer value=w534:u32)
            n210 = Unbundle By Name(w535) -> ("Tick Count"=w533:u32)
            n211 = call "SEQ Preview Queue.vi"("error in"=w538) -> ("error out"=w524:errorcluster, "SEQ Data"=w539:T18)  [unwired: 9 in]
            n212 = Unbundle By Name(w539) -> ("Air Sealing"=w527:bool, "Fluidic Process Done?"=w529:bool)
            n213 = Subtract(x=w534, y=w533) -> (x-y=w532:u32)
            n214 = Greater Or Equal?(x=w532, y=u32 60000) -> (x >= y?=w530:bool)
            n215 = Wait (ms)(milliseconds to wait=u32 100) -> ()  [unwired: 1 out]
            n216 = Bundle By Name(cluster=w535, "Chip Status.Air Sealing"=w527) -> (w528:T1)
            n217 = Or(x=w530, y=w529) -> (x .or. y?=w526:bool)
            n218 = case shown="False" w526 {
              tunnel: ["Air Tight Wait" "Homing"] -> w525
              frame False {
              }
              frame True {
              }
            }
            n219 = call "Enqueue.vi"("Error In"=w524, "State"=w525, "Queue in"=w536) -> ("Error Out"=w537:errorcluster)  [unwired: 7 in, 1 out]
          }
          frame "Homing" {
            n220 = call "Enqueue.vi"("Error In"=w543, "State"="Homing Wait", "Queue in"=w551) -> ("Error Out"=w548:errorcluster)  [unwired: 7 in, 1 out]
            n221 = call "Home.vi"("Error In"=w548) -> ("Error Out"=w547:errorcluster)  [unwired: 10 in]
            n222 = flat-sequence {
              tunnel: w547 -> [w553]
              tunnel: [w553] -> w546
              frame #0 {
                n223 = Wait (ms)(milliseconds to wait=u32 1000) -> ()  [unwired: 1 out]
              }
            }
            n224 = Tick Count (ms)() -> (millisecond timer value=w544:u32)
            n225 = Bundle By Name(cluster=w549, "Tick Count"=w544) -> (w545:T1)
          }
          frame "Homing Wait" {
            n226 = call "SEQ Preview Queue.vi"("error in"=w556) -> ("error out"=w555:errorcluster, "SEQ Data"=w557:T15)  [unwired: 9 in]
            n227 = Tick Count (ms)() -> (millisecond timer value=w565:u32)
            n228 = Unbundle By Name(w566) -> ("Tick Count"=w564:u32)
            n229 = Unbundle By Name(w557) -> ("Arrived?"=w554:bool)
            "Homing" <- w554
            n230 = Subtract(x=w565, y=w564) -> (x-y=w563:u32)
            n231 = Greater Or Equal?(x=w563, y=u32 120000) -> (x >= y?=w561:bool)
            n232 = Wait (ms)(milliseconds to wait=u32 100) -> ()  [unwired: 1 out]
            n233 = Bundle By Name(cluster=w566, "Chip Status.Homing"=w554) -> (w560:T1)
            n234 = Or(x=w561, y=w554) -> (x .or. y?=w559:bool)
            n235 = case shown="True" w559 {
              tunnel: ["Homing Wait" "Chip End"] -> w558
              frame False {
              }
              frame True {
              }
            }
            n236 = call "Enqueue.vi"("Error In"=w555, "State"=w558, "Queue in"=w567) -> ("Error Out"=w568:errorcluster)  [unwired: 7 in, 1 out]
          }
          frame "LED On" {
            n237 = call "Enqueue.vi"("Error In"=w578, "State"="Rotate U", "Queue in"=w577) -> ("Error Out"=w575:errorcluster)  [unwired: 7 in, 1 out]
            n238 = call "LED On.vi"("Error In"=w575, "Image Para"=T5 {"Marker"=enum."BF", "Power(Amp)"=55, "set shutter(s)"=0.05, "Cube"=enum."6"}) -> ("Error Out"=w573:errorcluster)  [unwired: 9 in]
            n239 = call "Rendezvous Acquire.vi"("Error In"=w573) -> ("Error Out"=w572:errorcluster)  [unwired: 10 in]
          }
          frame "Rotate U" {
            n240 = call "Enqueue.vi"("Error In"=w586, "State"="Change Expo", "Queue in"=w585) -> ("Error Out"=w583:errorcluster)  [unwired: 7 in, 1 out]
            n241 = call "Rotate U.vi"("Error In"=w583, "Cube"=enum16{"1", "2", "3", "4", "5", "6", "7", "8"}."6") -> ("Error Out"=w581:errorcluster)  [unwired: 9 in]
            n242 = call "Rendezvous Acquire.vi"("Error In"=w581) -> ("Error Out"=w580:errorcluster)  [unwired: 10 in]
          }
          frame "Change Expo" {
            n243 = call "Enqueue.vi"("Error In"=w594, "State"="Locating Wait", "Queue in"=w593) -> ("Error Out"=w591:errorcluster)  [unwired: 7 in, 1 out]
            n244 = call "Change Expo.vi"("Error In"=w591, "Expo(s)"=0.05) -> ("Error Out"=w589:errorcluster)  [unwired: 9 in]
            n245 = call "Rendezvous Acquire.vi"("Error In"=w589) -> ("Error Out"=w588:errorcluster)  [unwired: 10 in]
          }
          frame "Locating Wait" {
            n246 = call <vilib>:"Create Rendezvous.vi"("error in (no error)"=w598, "size (2)"=4, "name (unnamed)"="Acquire") -> ("error out"=w607:errorcluster, "rendezvous"=w605:T19)  [unwired: 2 in, 1 out]
            n247 = call <vilib>:"Wait at Rendezvous.vi"("error in (no error)"=w607, "ms timeout (-1)"=10000, "rendezvous"=w605) -> ("error out"=w606:errorcluster, "timed out"=w600:bool, "rendezvous out"=w604:T19)  [unwired: 2 in]
            n248 = call <vilib>:"Destroy Rendezvous.vi"("error in (no error)"=w606, "rendezvous"=w604) -> ("error out"=w599:errorcluster)  [unwired: 4 in, 1 out]
            n249 = case shown="False" w600 {
              tunnel: w599 -> [w612 _]
              tunnel: [w613 w616] -> w597
              tunnel: w596 -> [w610 _]
              frame False {
                n250 = flat-sequence {
                  tunnel: w612 -> [w614]
                  tunnel: [w614] -> w611
                  frame #0 {
                    n251 = Wait (ms)(milliseconds to wait=u32 200) -> ()  [unwired: 1 out]
                  }
                }
                n252 = call "Enqueue.vi"("Error In"=w611, "State"="Go Reference", "Queue in"=w610) -> ("Error Out"=w613:errorcluster)  [unwired: 7 in, 1 out]
              }
              frame True {
                n253 = xnode "Error Ring"() -> ("error out"=w616:errorcluster)
              }
            }
          }
          frame "Go Reference" {
            n254 = call "Enqueue.vi"("Error In"=w629, "State"="Go Reference Wait", "Queue in"=w628) -> ("Error Out"=w626:errorcluster)  [unwired: 7 in, 1 out]
            n255 = call "Go Reference.vi"("Error In"=w626) -> ("Error Out"=w625:errorcluster)  [unwired: 10 in]
            n256 = flat-sequence {
              tunnel: w625 -> [w631]
              tunnel: [w631] -> w624
              frame #0 {
                n257 = Wait (ms)(milliseconds to wait=u32 1000) -> ()  [unwired: 1 out]
              }
            }
            n258 = Tick Count (ms)() -> (millisecond timer value=w622:u32)
            n259 = Bundle By Name(cluster=w630, "Tick Count"=w622) -> (w623:T1)
          }
          frame "Go Reference Wait" {
            n260 = call "SEQ Preview Queue.vi"("error in"=w636) -> ("error out"=w635:errorcluster, "SEQ Data"=w637:T15)  [unwired: 9 in]
            n261 = Tick Count (ms)() -> (millisecond timer value=w644:u32)
            n262 = Unbundle By Name(w633) -> ("Tick Count"=w643:u32)
            n263 = Unbundle By Name(w637) -> ("Arrived?"=w634:bool)
            n264 = Subtract(x=w644, y=w643) -> (x-y=w642:u32)
            n265 = Greater Or Equal?(x=w642, y=u32 60000) -> (x >= y?=w640:bool)
            n266 = Wait (ms)(milliseconds to wait=u32 100) -> ()  [unwired: 1 out]
            n267 = Or(x=w640, y=w634) -> (x .or. y?=w639:bool)
            n268 = case shown="True" w639 {
              tunnel: ["Go Reference Wait" "Locating Triangle"] -> w638
              frame False {
              }
              frame True {
              }
            }
            n269 = call "Enqueue.vi"("Error In"=w635, "State"=w638, "Queue in"=w645) -> ("Error Out"=w646:errorcluster)  [unwired: 7 in, 1 out]
          }
          frame "Locating Triangle" {
            n270 = Unbundle By Name(w659) -> ("Folder Path"=w658:path)
            n271 = call "Enqueue.vi"("Error In"=w664, "State"="Locating Triangle Wait", "Queue in"=w663) -> ("Error Out"=w654:errorcluster)  [unwired: 7 in, 1 out]
            n272 = Build Path(base path=w658, name or relative path="Locating Chip") -> (appended path=w656:path)
            n273 = call "Create Folder.vi"("error in"=w654, "Path in"=w656) -> ("error out"=w653:errorcluster, "Path out"=w655:path)  [unwired: 8 in]
            n274 = Bundle By Name(cluster=T8 {"Image Path"=path "", "Start Offset"=0, "Template Path"=path "", "Disable Fine Search"=FALSE, "ROI"={"Global Rectangle"=[], "Contours"=[]}} ("Match Data"), "Template Path"=path "C:/MiCareo/MiSelectMiControl/PARAMETER/IMAGE/20180613.png" ("File Path"), "Start Offset"=0, "Disable Fine Search"=TRUE, "Image Path"=w655, "ROI"=T7 {"Global Rectangle"=[0, 0, 2560, 2160], "Contours"=[{"ID"=enum."External", "Type"=3, "Coordinates"=[0, 0, 2560, 2160, 0]}]}) -> (w650:T8)
            n275 = Tick Count (ms)() -> (millisecond timer value=w660:u32)
            n276 = Bundle By Name(cluster=w659, "Tick Count"=w660) -> (w661:T1)
            n277 = call "Match Pattern.vi"("Error In"=w653, "Match Data"=w650) -> ("Error Out"=w666:errorcluster)  [unwired: 9 in]
            n278 = flat-sequence {
              tunnel: w666 -> [w671]
              tunnel: [w671] -> w665
              frame #0 {
                n279 = Wait (ms)(milliseconds to wait=u32 1000) -> ()  [unwired: 1 out]
              }
            }
          }
          frame "Locating Triangle Wait" {
            n280 = call "SEQ Preview Queue.vi"("error in"=w675) -> ("error out"=w674:errorcluster, "SEQ Data"=w676:T20)  [unwired: 9 in]
            n281 = Tick Count (ms)() -> (millisecond timer value=w683:u32)
            n282 = Unbundle By Name(w672) -> ("Tick Count"=w682:u32)
            n283 = Unbundle By Name(w676) -> ("Match Done?"=w673:bool)
            n284 = Subtract(x=w683, y=w682) -> (x-y=w681:u32)
            n285 = Greater Or Equal?(x=w681, y=u32 180000) -> (x >= y?=w679:bool)
            n286 = Wait (ms)(milliseconds to wait=u32 100) -> ()  [unwired: 1 out]
            n287 = Or(x=w679, y=w673) -> (x .or. y?=w678:bool)
            n288 = case shown="True" w678 {
              tunnel: ["Locating Triangle Wait" "Locating Flower"] -> w677
              frame False {
              }
              frame True {
              }
            }
            n289 = call "Enqueue.vi"("Error In"=w674, "State"=w677, "Queue in"=w684) -> ("Error Out"=w685:errorcluster)  [unwired: 7 in, 1 out]
          }
          frame "Locating Flower" {
            n290 = Unbundle By Name(w698) -> ("Folder Path"=w696:path)
            n291 = call "Enqueue.vi"("Error In"=w704, "State"="Locating Flower Wait", "Queue in"=w703) -> ("Error Out"=w695:errorcluster)  [unwired: 7 in, 1 out]
            n292 = Build Path(base path=w696, name or relative path="Locating Chip") -> (appended path=w693:path)
            n293 = call "Create Folder.vi"("error in"=w695, "Path in"=w693) -> ("error out"=w694:errorcluster, "Path out"=w692:path)  [unwired: 8 in]
            n294 = Bundle By Name(cluster=T8 {"Image Path"=path "", "Start Offset"=0, "Template Path"=path "", "Disable Fine Search"=FALSE, "ROI"={"Global Rectangle"=[], "Contours"=[]}} ("Match Data"), "Template Path"=path "C:/MiCareo/MiSelectMiControl/PARAMETER/IMAGE/Chip/Chip20160427.png" ("File Path"), "Start Offset"=0, "Disable Fine Search"=FALSE, "Image Path"=w692, "ROI"=T7 {"Global Rectangle"=[1030, 830, 1530, 1330], "Contours"=[{"ID"=enum."External", "Type"=3, "Coordinates"=[1030, 830, 1530, 1330, 0]}]}) -> (w689:T8)
            n295 = Tick Count (ms)() -> (millisecond timer value=w700:u32)
            n296 = Bundle By Name(cluster=w698, "Tick Count"=w700) -> (w701:T1)
            n297 = call "Match Pattern.vi"("Error In"=w694, "Match Data"=w689) -> ("Error Out"=w706:errorcluster)  [unwired: 9 in]
            n298 = flat-sequence {
              tunnel: w706 -> [w710]
              tunnel: [w710] -> w705
              frame #0 {
                n299 = Wait (ms)(milliseconds to wait=u32 1000) -> ()  [unwired: 1 out]
              }
            }
          }
          frame "Locating Flower Wait" {
            n300 = call "SEQ Preview Queue.vi"("error in"=w715) -> ("error out"=w714:errorcluster, "SEQ Data"=w716:T20)  [unwired: 9 in]
            n301 = Unbundle By Name(w712) -> ("Tick Count"=w722:u32)
            n302 = Unbundle By Name(w716) -> ("Match Done?"=w713:bool)
            n303 = Tick Count (ms)() -> (millisecond timer value=w723:u32)
            n304 = Subtract(x=w723, y=w722) -> (x-y=w721:u32)
            n305 = Greater Or Equal?(x=w721, y=u32 180000) -> (x >= y?=w719:bool)
            n306 = Or(x=w719, y=w713) -> (x .or. y?=w718:bool)
            n307 = case shown="True" w718 {
              tunnel: ["Locating Flower Wait" "Locating Score"] -> w717
              frame False {
              }
              frame True {
              }
            }
            n308 = Wait (ms)(milliseconds to wait=u32 100) -> ()  [unwired: 1 out]
            n309 = call "Enqueue.vi"("Error In"=w714, "State"=w717, "Queue in"=w724) -> ("Error Out"=w711:errorcluster)  [unwired: 7 in, 1 out]
          }
          frame "Locating Score" {
            n310 = call "Enqueue.vi"("Error In"=w737, "State"="LED Off", "Queue in"=w736) -> ("Error Out"=w731:errorcluster)  [unwired: 7 in, 1 out]
            n311 = call "SEQ Preview Queue.vi"("error in"=w731) -> ("error out"=w730:errorcluster, "SEQ Data"=w734:T20)  [unwired: 9 in]
            n312 = Unbundle By Name(w734) -> ("Match Score"=w733:dbl)
            n313 = Greater?(x=w733, y=300.0) -> (0:w728:bool)
            n314 = Bundle By Name(cluster=w738, "Chip Status.Locating"=w728) -> (w729:T1)
          }
          frame "LED Off" {
            n315 = call "Enqueue.vi"("Error In"=w743, "State"="Chip End", "Queue in"=w742) -> ("Error Out"=w740:errorcluster)  [unwired: 7 in, 1 out]
            n316 = call "LED Off.vi"("Error In"=w740) -> ("Error Out"=w739:errorcluster)  [unwired: 10 in]
          }
          frame "Chip End" {
            n317 = call <vilib>:"Unset Busy.vi"("error in (no error)"=w747) -> ("error out"=w746:errorcluster)  [unwired: 10 in]
            n318 = Unbundle By Name(w748) -> ("Chip Status.Homing"=w745:bool)
            n319 = case shown="False" w745 {
              tunnel: w746 -> [w756 w763]
              tunnel: [w755 w762] -> w750
              tunnel: w749 -> [w754 w761]
              frame True {
                n320 = Bundle By Name(cluster=T3 {"State"="", "Data"=variant} ("event data"), "State"="Done") -> (w752:T3)
                n321 = Generate User Event(user event=w754, event data cluster=w752, error in=w756) -> (error out=w755:errorcluster)  [unwired: 1 in, 1 out]
              }
              frame False {
                n322 = Bundle By Name(cluster=T3 {"State"="", "Data"=variant} ("event data"), "State"="Abort") -> (w759:T3)
                n323 = Generate User Event(user event=w761, event data cluster=w759, error in=w763) -> (error out=w762:errorcluster)  [unwired: 1 in, 1 out]
                n324 = One Button Dialog(message="Chip Initialization Fail. Please Click \"Abort\".") -> ()  [unwired: 1 in, 1 out]
              }
            }
          }
          frame "------Close------" {
          }
          frame "Close" {
            n325 = Release Queue(queue=w769, error in (no error)=w770) -> (error out=w768:errorcluster)  [unwired: 1 in, 2 out]
          }
        }
      }
      n326 = while {
        tunnel: w9 -> [w25]
        tunnel: [w19] -> w12
        tunnel: w4 -> [w23]
        tunnel: w7 -> [w22]
        tunnel: w3 -> [w21]
        stop <- w24 stop-if-true
        n327 = event shown="[2] \"Start\": Value Change" {
          selector: w23 -> [_ _ _ _ w85 w91]
          dyn-events: _ -> [_ _ _ _ _ _]
          timeout: _ -> [_ _ _ _ _ _]
          tunnel: w25 -> [w26 w28 w67 w74 w84 w98]
          tunnel: [w26 w29 w66 w73 w78 w93] -> w20
          tunnel: [_ _ _ _ TRUE TRUE] -> w24
          tunnel: w22 -> [_ _ w65 w72 w82 w97]
          tunnel: w21 -> [_ _ _ _ w79 w90]
          tunnel: [_ enum16{"None", "Write"}."None" ("Action") enum16{"None", "Write"}."None" ("Action") enum16{"None", "Write"}."Write" ("Action") enum16{"None", "Write"}."Write" ("Action") enum16{"None", "Write"}."Write" ("Action")] -> w18
          tunnel: [_ _ w58 w68 w76 w88] -> w16
          event Timeout {
            n328 = event-data() -> ()  [unwired: 1 in, 1 out]
          }
          event User Event {
            n329 = event-data() -> ("State"=w31:string, "Data"=w30:variant)  [unwired: 1 in]
            n330 = case shown="\"Start\"" w31 {
              selector: w31 -> [w32 _ _ _ _]
              tunnel: w30 -> [_ _ _ _ _]
              tunnel: [w35 w40 w45 w50 w55] -> w29
              tunnel: w28 -> [w35 w40 w45 w50 w55]
              frame "Typo", Default {
                n331 = Concatenate Strings("Typo: " ("string"), w32) -> (w33:string)
                n332 = One Button Dialog(message=w33) -> ()  [unwired: 1 in, 1 out]
              }
              frame "Start" {
                n333 = property on="Abort" class="Bool"("Visible"=TRUE) -> ()  [unwired: 2 in, 2 out]
                n334 = property on="Start" class="Bool"("Visible"=TRUE) -> ()  [unwired: 2 in, 2 out]
                n335 = property on="Next" class="Bool"("Visible"=FALSE) -> ()  [unwired: 2 in, 2 out]
                n336 = property on="Done" class="Bool"("Visible"=FALSE) -> ()  [unwired: 2 in, 2 out]
              }
              frame "Next" {
                n337 = property on="Abort" class="Bool"("Visible"=TRUE) -> ()  [unwired: 2 in, 2 out]
                n338 = property on="Start" class="Bool"("Visible"=FALSE) -> ()  [unwired: 2 in, 2 out]
                n339 = property on="Next" class="Bool"("Visible"=TRUE) -> ()  [unwired: 2 in, 2 out]
                n340 = property on="Done" class="Bool"("Visible"=FALSE) -> ()  [unwired: 2 in, 2 out]
              }
              frame "Done" {
                n341 = property on="Abort" class="Bool"("Visible"=TRUE) -> ()  [unwired: 2 in, 2 out]
                n342 = property on="Start" class="Bool"("Visible"=FALSE) -> ()  [unwired: 2 in, 2 out]
                n343 = property on="Next" class="Bool"("Visible"=FALSE) -> ()  [unwired: 2 in, 2 out]
                n344 = property on="Done" class="Bool"("Visible"=TRUE) -> ()  [unwired: 2 in, 2 out]
              }
              frame "Abort" {
                n345 = property on="Abort" class="Bool"("Visible"=TRUE) -> ()  [unwired: 2 in, 2 out]
                n346 = property on="Start" class="Bool"("Visible"=FALSE) -> ()  [unwired: 2 in, 2 out]
                n347 = property on="Next" class="Bool"("Visible"=FALSE) -> ()  [unwired: 2 in, 2 out]
                n348 = property on="Done" class="Bool"("Visible"=FALSE) -> ()  [unwired: 2 in, 2 out]
              }
            }
          }
          event "Start": Value Change {
            w63 = cluster{"Operator":string, "Experiment":string} {"Operator"="", "Experiment"=""}  # User Info
            n349 = event-data() -> ("CtlRef"=w59:refnum<vi>)  [unwired: 1 in]
            n350 = property class="Bool"(reference=w59) -> ("Label.Text"=w58:string)  [unwired: 1 in, 2 out]
            n351 = Bundle By Name(cluster=w63, "Operator"="Operator", "Experiment"="Experiment") -> (w62:cluster{"Operator":string, "Experiment":string})
            n352 = To Variant(anything=w62) -> (Variant=w61:variant)
            n353 = call "Enqueue.vi"("Error In"=w67, "Data"=w61, "State"="Check Empty", "Queue in"=w65) -> ("Error Out"=w66:errorcluster)  [unwired: 6 in, 1 out]
          }
          event "Next": Value Change {
            n354 = event-data() -> ("CtlRef"=w69:refnum<vi>)  [unwired: 1 in]
            n355 = property class="Bool"(reference=w69) -> ("Label.Text"=w68:string)  [unwired: 1 in, 2 out]
            n356 = call "Enqueue.vi"("Error In"=w74, "State"="Homing", "Queue in"=w72) -> ("Error Out"=w73:errorcluster)  [unwired: 7 in, 1 out]
          }
          event "Abort": Value Change {
            n357 = event-data() -> ("CtlRef"=w77:refnum<vi>)  [unwired: 1 in]
            n358 = property class="Bool"(reference=w77) -> ("Label.Text"=w76:string)  [unwired: 1 in, 2 out]
            n359 = call "Enqueue.vi"("Error In"=w84, "State"="Close", "Queue in"=w82) -> ("Error Out"=w83:errorcluster)  [unwired: 7 in, 1 out]
            n360 = Unregister For Events(event registration refnum=w85, error in=w83) -> (error out=w80:errorcluster)
            n361 = Destroy User Event(user event=w79, error in=w80) -> (error out=w78:errorcluster)
          }
          event "Done": Value Change {
            n362 = event-data() -> ("CtlRef"=w89:refnum<vi>)  [unwired: 1 in]
            n363 = property class="Bool"(reference=w89) -> ("Label.Text"=w88:string)  [unwired: 1 in, 2 out]
            n364 = call "Enqueue.vi"("Error In"=w98, "State"="Close", "Queue in"=w97) -> ("Error Out"=w95:errorcluster)  [unwired: 7 in, 1 out]
            n365 = Unregister For Events(event registration refnum=w91, error in=w95) -> (error out=w94:errorcluster)
            n366 = Destroy User Event(user event=w90, error in=w94) -> (error out=w93:errorcluster)
          }
        }
        n367 = call "Log.vi"("Action"=w18, "error in"=w20, "State"=w16, "Page Name"="Initialize") -> ("error out"=w19:errorcluster)  [unwired: 7 in]
      }
      n368 = Merge Errors(w12, w11) -> (w6:errorcluster)
    }
    frame Error {
    }
  }
  "error out" <- w1
